vi "WaitForProgramLoad.vi"(0 "Universal Robot.lvclass in":refnum<class "Universal Robot.lvclass">, 1 "program in":string, 5 "error in (no error)":errorcluster, 8 "timeout (ms)":u32=5000) -> (14 "Universal Robot.lvclass out":refnum<class "Universal Robot.lvclass">, 19 "error out":errorcluster)   [LabVIEW 2019, in "Universal Robot.lvclass"]
uses:
  Universal Robot.lvclass
panel:
  out "Load Time":u32
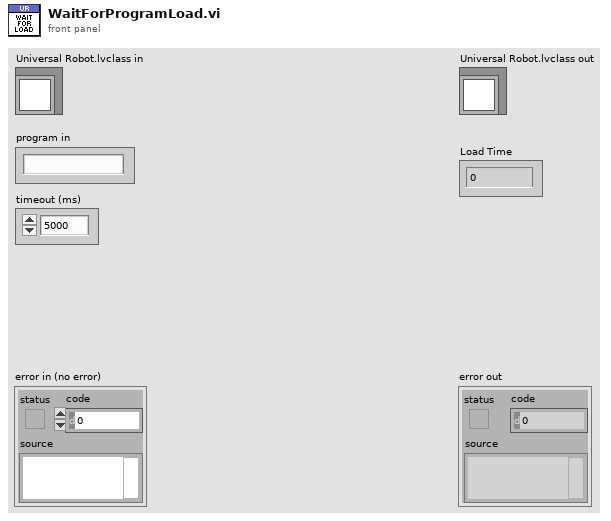
[diagram p1: front panel]
types:
  T1 = typedef "Universal Robot.lvclass/ProgramStatus.ctl" = cluster{"Loaded Program":string, "Valid Program":bool, "Program State":T2, "Running":bool}
  T2 = typedef "Universal Robot.lvclass/ProgramState.ctl" = enum16{"STOPPED", "PLAYING", "PAUSE"}
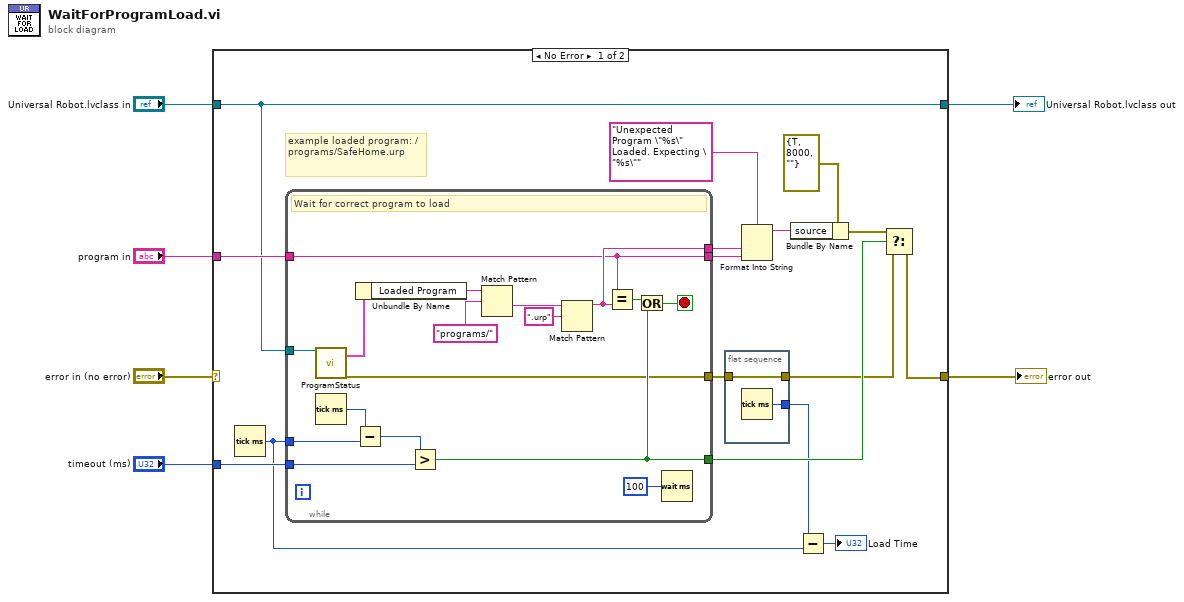
[diagram p0: block diagram]
diagram:
  n1 = case shown="No Error" "error in (no error)" {
    selector: "error in (no error)" -> [_ w43]
    tunnel: [w17 w43] -> w5
    tunnel: "Universal Robot.lvclass in" -> [w13 w42]
    tunnel: [w13 w42] -> w3
    tunnel: "program in" -> [w22 _]
    tunnel: "timeout (ms)" -> [w12 _]
    frame No Error {
      # "example loaded program: /programs/SafeHome.urp"
      n2 = Tick Count (ms)() -> (millisecond timer value=w9:u32)
      n3 = while {
        tunnel: w9 -> [w41]
        tunnel: [w25] -> w11
        tunnel: [w40] -> w18
        tunnel: w22 -> [w30]
        tunnel: [w31] -> w21
        tunnel: [w30] -> w20
        tunnel: w13 -> [w29]
        tunnel: w12 -> [w28]
        stop <- w39 stop-if-true
        # "Wait for correct program to load"
        n4 = call-dynamic "ProgramStatus.vi"("Universal Robot.lvclass in"=w29) -> ("Program Status"=w33:T1, "error out"=w25:errorcluster)  [unwired: 16 in, 1 out]
        n5 = Tick Count (ms)() -> (millisecond timer value=w27:u32)
        n6 = Subtract(x=w27, y=w41) -> (x-y=w38:u32)
        n7 = Unbundle By Name(w33) -> ("Loaded Program"=w37:string)
        n8 = Greater?(x=w38, y=w28) -> (0:w40:bool)
        n9 = Match Pattern(string=w37, regular expression="programs/") -> (after substring=w35:string)  [unwired: 1 in, 3 out]
        n10 = Match Pattern(string=w35, regular expression=".urp") -> (before substring=w31:string)  [unwired: 1 in, 3 out]
        n11 = Equal?(x=w30, y=w31) -> (x = y?=w32:bool)
        n12 = Or(x=w32, y=w40) -> (x .or. y?=w39:bool)
        n13 = Wait (ms)(milliseconds to wait=u32 100) -> ()  [unwired: 1 out]
      }
      n14 = flat-sequence {
        tunnel: w11 -> [w24]
        tunnel: [w24] -> w10
        tunnel: [w23] -> w8
        frame #0 {
          n15 = Tick Count (ms)() -> (millisecond timer value=w23:u32)
        }
      }
      n16 = Format Into String(format string="Unexpected Program \"%s\" Loaded. Expecting \"%s\"", w21, w20) -> (resulting string=w15:string)  [unwired: 2 in, 1 out]
      n17 = Bundle By Name(cluster=errorcluster {"status"=TRUE, "code"=8000, "source"=""} ("error constant"), "source"=w15) -> (w14:errorcluster)
      n18 = Subtract(x=w8, y=w9) -> (x-y=→"Load Time":u32)
      n19 = Select(t=w14, s=w18, f=w10) -> (s? t:f=w17:errorcluster)
    }
    frame Error {
    }
  }
  "error out" <- w5
  "Universal Robot.lvclass out" <- w3
